vi "Fpga-Uart-State-Machine.vi"(5 "reset_rtl":bool, 6 "TX FIFO In":refnum<k21>="HT-UART_TX", 7 "RXD Pin In":refnum<k21>="UserRTL_d_microblaze_wrapper\\uart_rtl_rxd", 8 "RX FIFO In":refnum<k21>="TH-UART_RX", 9 "TXD Pin In":refnum<k21>="UserRTL_d_microblaze_wrapper\\uart_rtl_txd", 10 "Baud Rate":u32(ring)=128000 items=["110"=110, "300"=300, "1200"=1200, "2400"=2400, "4800"=4800, "9600"=9600, "19200"=19200, "38400"=38400, "57600"=57600, "115200"=115200, "128000"=128000, "230400"=230400, "460800"=460800, "921600"=921600], 11 "FPGA Clock Rate (MHz)":u32=100) -> ()   [LabVIEW 2017]
uses:
  <vilib>/Platform/TimedLoop/XDataNode/timing_clust.ctl
  <vilib>/Platform/TimedLoop/XDataNode/nitl_modes.ctl
  <vilib>/Platform/TimedLoop/XDataNode/wakeup.ctl
  UART.RX.States.2.ctl
  UART.RX.States.ctl
  <vilib>/rvi/Emulation/niFpgaSctlEmulationGetInTimedLoop.vi
  <vilib>/rvi/Emulation/niFpgaEmulationReportErrorSimple.vi
  <vilib>/rvi/Emulation/niFpgaGetClockAttributes.vi
  <vilib>/rvi/Emulation/niFpgaCriticalErrorInLSC.vi
  <vilib>/rvi/eio/common/nirviEmuTemplateMethod_errors.vi
  <vilib>/rvi/DataTransferAndStorage/Container/Common/niFpgaContainerExecOnDevCompGetState.vi
  <vilib>/rvi/Emulation/niFpgaEmulationIsFPGAContextNoSignature.vi
  <vilib>/rvi/errors/niFpgaSetErrorForExecOnDevCompSimple.vi
  <vilib>/rvi/eio/common/nirviEmuReportErrorAndStop.vi
  <vilib>/rvi/DataTransferAndStorage/Container/Common/niFpgaContainerGetUniqueNameForEmu.vi
  <vilib>/rvi/FIFO/Fifo_Resource/nirvififoEmulationSetSize.vi
  <vilib>/rvi/FIFO/Fifo_Resource/nirviFifoEmulationQueueMgr.vi
  <instcachedir>/0/nirviFifoEmulationQueueMgr_E5CAEC123FF24DC58D834DCA3CDAA9B5.lvgen/nirviFifoEmulationQueueMgr_E5CAEC123FF24DC58D834DCA3CDAA9B5_004.vi
  <vilib>/rvi/FIFO/Fifo_Resource/nirvififoEmulationDetermineInputValidOut.vi
  <vilib>/rvi/FIFO/Fifo_Resource/nirvififoEmulationCreateLock.vi
  <vilib>/rvi/Emulation/niFpgaProcessEmulError.vi
  <vilib>/rvi/FIFO/Fifo_Resource/nirvififoEmulationObtainLock.vi
  <vilib>/rvi/FIFO/Fifo_Resource/nirvififoEmulationReleaseLock.vi
  <vilib>/rvi/occurrence/nirviWaitOnOccurrenceBase.vi
  <vilib>/rvi/errors/nirviReportUnexpectedCaseInternalError.vi
  <vilib>/rvi/errors/nirviReportUnexpectedCaseInternalError (U32).vi
  <vilib>/Utility/error.llb/Clear Errors.vi
  <vilib>/rvi/interface/RandomDataEmulation/niFpgaRandomDataHandleErrors.vi
  <vilib>/Platform/TimedLoop/XDataNode/XDataNode.xnode
  <vilib>/eio/EIONode/EIONode.xnode
  <vilib>/rvi/DataTransferAndStorage/Container/XNode/niFpgaContainer.xnode
  <vilib>/rvi/FIFO/Fifo_Resource/niFpgaFifoEmulationRefIn.vi
  <vilib>/Platform/TimedLoop/XDataNode/XDNodeRunTimeDep.lvlib
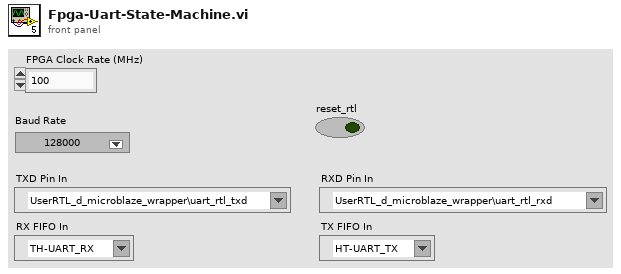
[diagram p1: front panel]
types:
  T1 = typedef "XDNodeRunTimeDep.lvlib/timing_clust.ctl" = cluster{"Expected End [f-1]":u64, "Actual End [f-1]":u64, "Finished Late? [f-1]":bool, "Expected End [i-1]":u64, "Actual End [i-1]":u64, "Finished Late? [i-1]":bool, "Expected Start [i]":u64, "Actual Start [i]":u64, "Expected Start [f]":u64, "Actual Start [f]":u64, "Source Name":string, "Structure Name":string, "Period":i64, "Deadline":i64, "Offset":i64, "Start":i64, "Priority":i32, "Timeout":i32, "Mode":T2, "Wakeup Reason":T3, "Error":errorcluster, "Source Type":string, "Secondary Source Type":string, "Global End Time":u64, "Global Start Time":u64, "Frame Duration":u64, "Iteration Duration":u64, "Assigned CPU":i32, "I/O Scan Engine Mode":u32}
  T2 = typedef "XDNodeRunTimeDep.lvlib/nitl_modes.ctl" = enum32{"No Change", "Process missed periods, maintain original phase", "Discard missed periods, maintain original phase", "Process missed periods, ignore original phase", "Discard missed periods, ignore original phase"}
  T3 = typedef "XDNodeRunTimeDep.lvlib/wakeup.ctl" = enum32{"Normal", "Aborted", "Asynchronous wakeup", "Timing source error", "Timed loop error", "Timeout"}
  T4 = typedef "UART.RX.States.2.ctl" = enum16{"No-Wait", "Wait-Half", "Wait-Full", "Wait-One-and-a-Half"}
  T5 = typedef "UART.RX.States.ctl" = enum16{"Read-StartBit", "Read-DataBits", "Read-Parity", "Read-StopBit", "Shift"}
  T6 = enum16{"Wait.for.New", "Send.StartBit", "Send.DataBits", "Send.Parity", "Send.StopBit"}
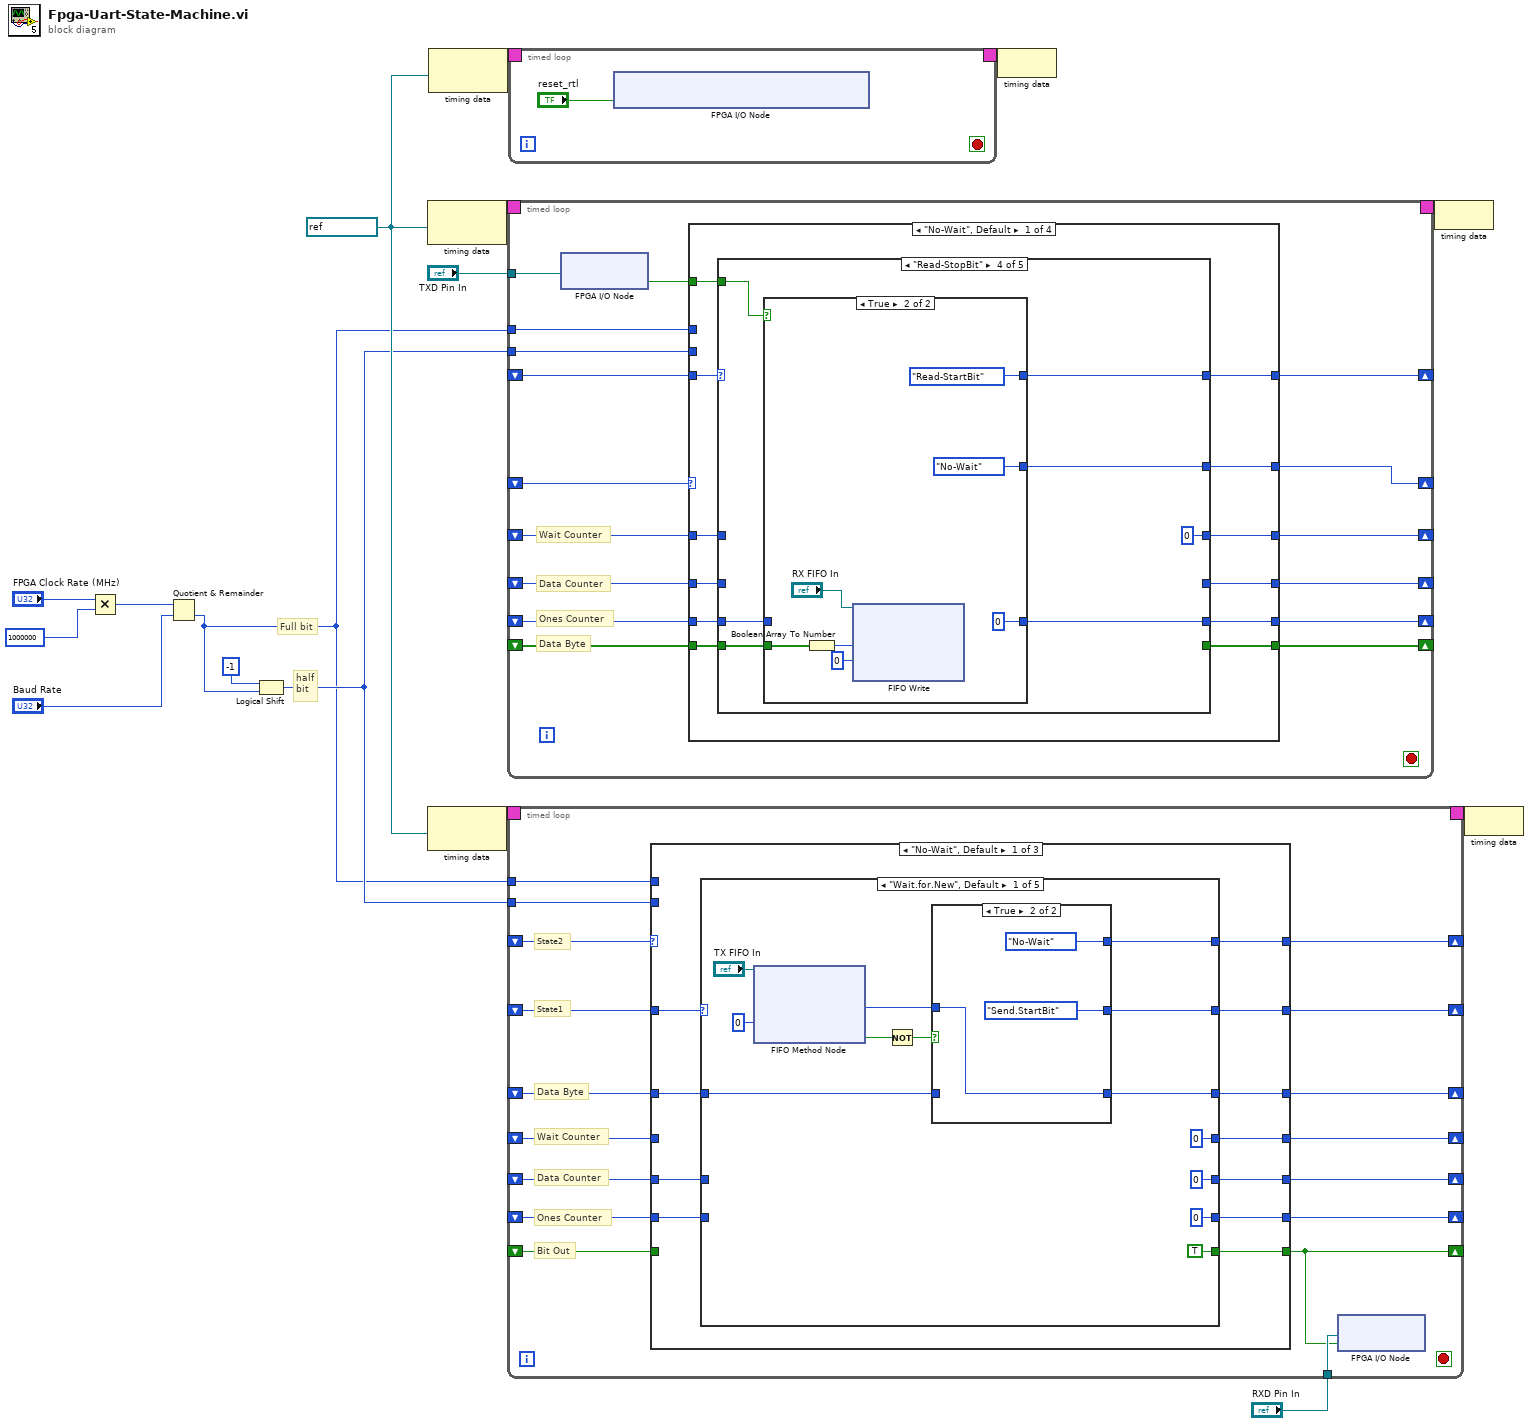
[diagram p0: block diagram]
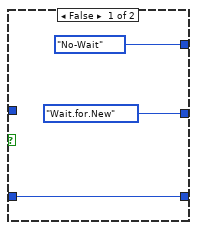
[diagram p2: hidden frame]
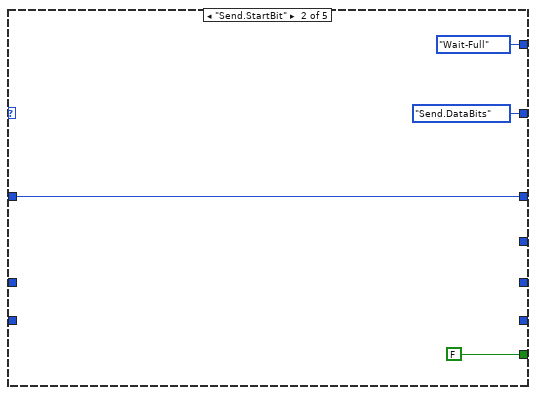
[diagram p3: hidden frame]
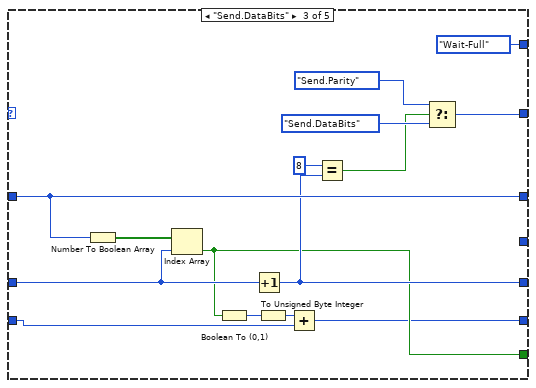
[diagram p4: hidden frame]
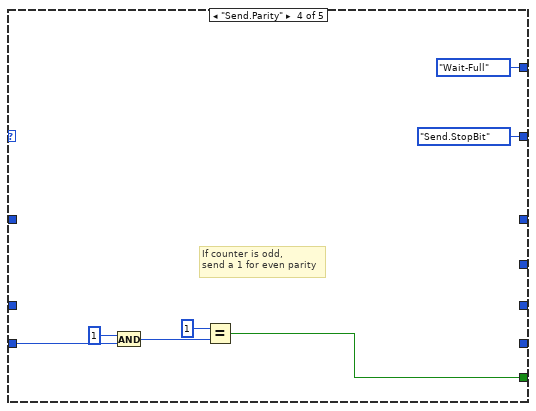
[diagram p5: hidden frame]
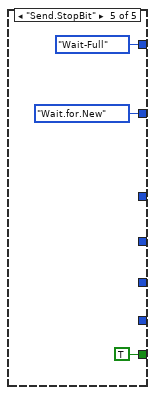
[diagram p6: hidden frame]
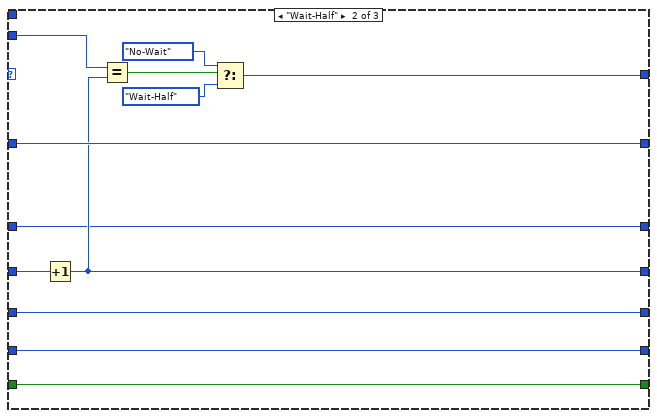
[diagram p7: hidden frame]
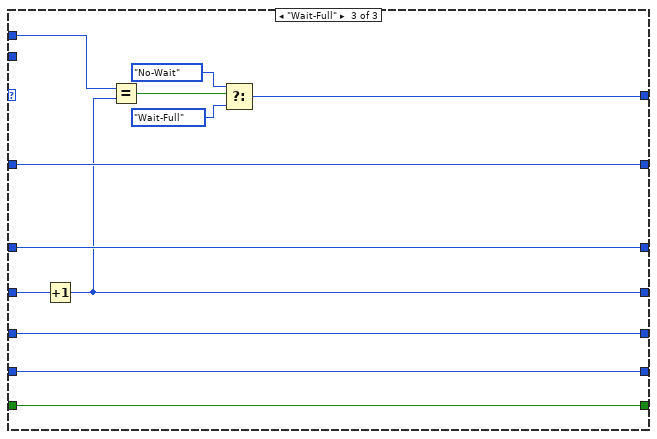
[diagram p8: hidden frame]
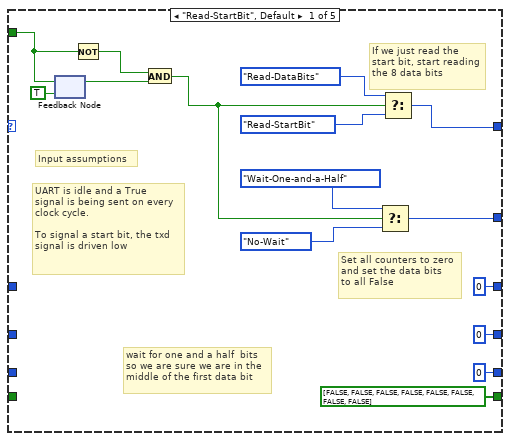
[diagram p9: hidden frame]
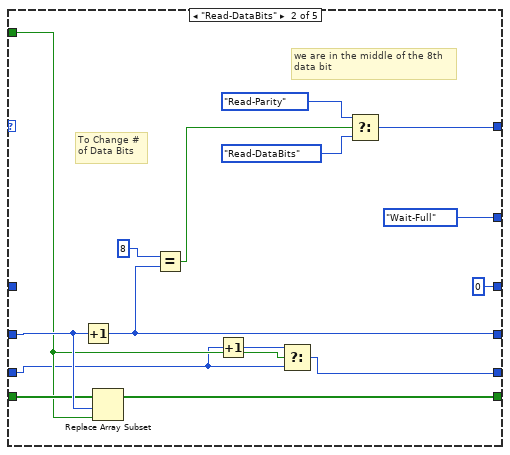
[diagram p10: hidden frame]
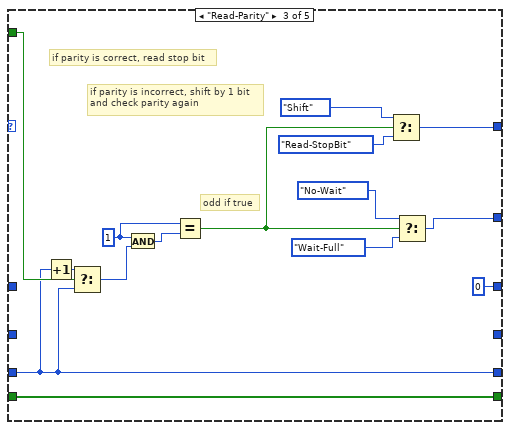
[diagram p11: hidden frame]
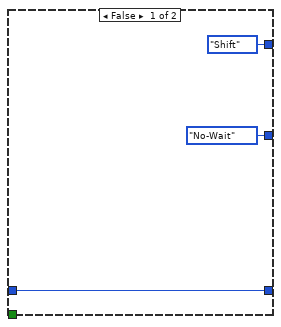
[diagram p12: hidden frame]
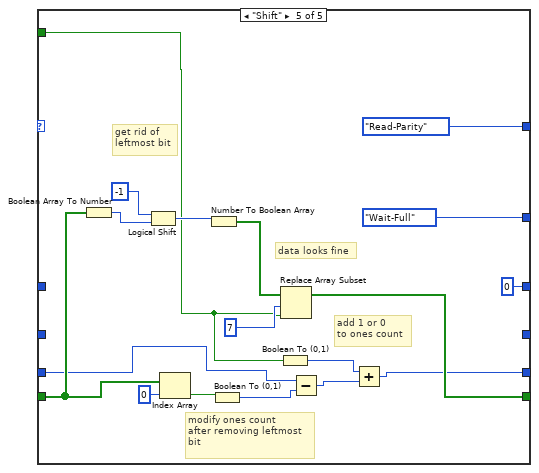
[diagram p13: hidden frame]
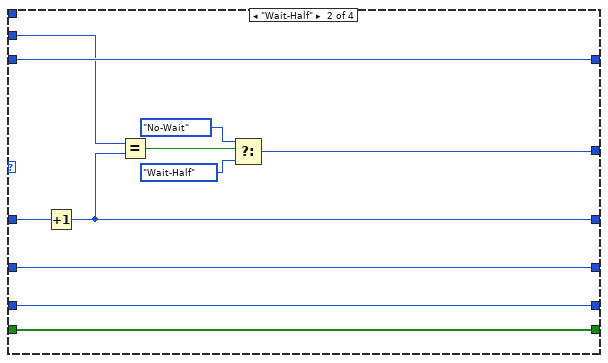
[diagram p14: hidden frame]
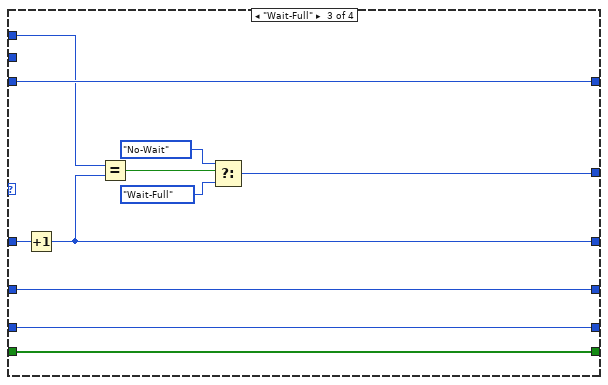
[diagram p15: hidden frame]
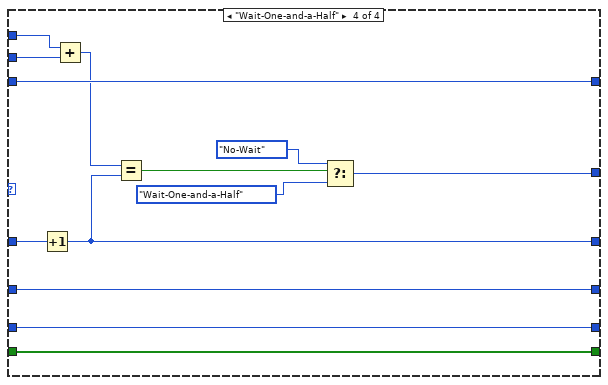
[diagram p16: hidden frame]
diagram:
  w3 = refnum<k21> "100MHz" ("Source Name")
  # "half\nbit"
  # "Full bit"
  n1 = Multiply(x="FPGA Clock Rate (MHz)", y=u32 1000000) -> (x*y=w15:u32)
  n2 = Quotient & Remainder(x=w15, y="Baud Rate") -> (floor(x/y)=w1:u32)  [unwired: 1 out]
  n3 = Logical Shift(y=i16 -1, x=w1) -> (x << y=w2:u32)
  n4 = node-c288(w3) -> (w10:T1)
  n5 = node-c288(w3) -> (w6:T1)
  n6 = node-c288(w3) -> (w12:T1)
  n7 = timed-loop {
    timing: w10 -> [_]
    timing-out: [_] -> w9
    shift-right: [w31] -> _
    shift-left: _ -> [w32]
    shift-right: [w29] -> _
    shift-left: _ -> [w30]
    shift-right: [w26] -> _
    shift-left: _ -> [w28]
    shift-right: [w25] -> _
    shift-left: _ -> [w27]
    tunnel: w1 -> [w24]
    tunnel: w2 -> [w23]
    shift-right: [w22] -> _
    shift-left: _ -> [w21]
    shift-right: [w19] -> _
    shift-left: _ -> [w20]
    tunnel: "TXD Pin In" -> [w18]
    stop <- _ stop-if-true
    # "Data Byte"
    # "Ones Counter"
    # "Data Counter"
    # "Wait Counter"
    n8 = xnode "FPGA I/O Node"("FPGA I/O In"=w18) -> ("I/O Item"=w17:bool)  [unwired: 1 out]
    n9 = case shown="\"No-Wait\", Default" w30 {
      tunnel: w32 -> [w40 w129 w138 w151]
      tunnel: w17 -> [w33 _ _ _]
      tunnel: [w39 w129 w138 w151] -> w31
      tunnel: [w38 w130 w142 w155] -> w29
      tunnel: w28 -> [w44 w135 w143 w156]
      tunnel: w27 -> [w43 w128 w141 w154]
      tunnel: [w37 w134 w140 w153] -> w26
      tunnel: [w36 w128 w141 w154] -> w25
      tunnel: w24 -> [_ _ w137 w149]
      tunnel: w23 -> [_ w126 _ w148]
      tunnel: [w34 w127 w139 w152] -> w22
      tunnel: w21 -> [w42 w127 w139 w152]
      tunnel: w20 -> [w41 w125 w136 w150]
      tunnel: [w35 w125 w136 w150] -> w19
      frame "No-Wait", Default {
        n10 = case shown="\"Read-StopBit\"" w40 {
          tunnel: w33 -> [w56 w64 w89 w95 w111]
          tunnel: [w55 w65 w85 w93 UART.RX.States."Read-Parity"] -> w39
          tunnel: [w49 UART.RX.States.2."Wait-Full" w80 w94 UART.RX.States.2."Wait-Full"] -> w38
          tunnel: w44 -> [_ _ _ _ _]
          tunnel: w43 -> [_ w73 _ _ _]
          tunnel: [u32 0 ("Wait Counter") u32 0 ("Wait Counter") u32 0 ("Wait Counter") u32 0 ("Wait Counter") u32 0 ("Wait Counter")] -> w37
          tunnel: [u32 0 ("Data Counter") w70 _ _ _] -> w36
          tunnel: [bool[] [FALSE, FALSE, FALSE, FALSE, FALSE, FALSE, FALSE, FALSE] w71 w78 _ w117] -> w34
          tunnel: w42 -> [_ w72 w78 w96 w116]
          tunnel: w41 -> [_ w63 w76 w91 w114]
          tunnel: [u32 0 ("Data Counter") w61 w76 w92 w109] -> w35
          frame "Read-StartBit", Default {
            # "Set all counters to zero\nand set the data bits\nto all False"
            # "wait for one and a half  bits\nso we are sure we are in the\nmiddle of the first data bit"
            # "If we just read the \nstart bit, start reading\nthe 8 data bits"
            # "UART is idle and a True\nsignal is being sent on every\nclock cycle.\n\nTo signal a start bit, the txd\nsignal is driven low"
            # "Input assumptions"
            n11 = feedback #1(TRUE ("d_microblaze_i\\uart_rtl_txd")) -> (w59:bool)
            n12 = feedback-in #1(w56) -> ()
            n13 = Not(x=w56) -> (.not. x?=w58:bool)
            n14 = And(x=w58, y=w59) -> (x .and. y?=w52:bool)
            n15 = Select(t=UART.RX.States.2."Wait-One-and-a-Half", s=w52, f=UART.RX.States.2."No-Wait") -> (s? t:f=w49:T4)
            n16 = Select(t=UART.RX.States."Read-DataBits", s=w52, f=UART.RX.States."Read-StartBit") -> (s? t:f=w55:T5)
          }
          frame "Read-DataBits" {
            # "we are in the middle of the 8th\ndata bit"
            # "To Change #\nof Data Bits"
            n17 = Increment(x=w73) -> (x+1=w70:u32)
            n18 = Replace Array Subset(array=w72, new element=w64, index=w73) -> (w71:bool[])
            n19 = Equal?(x=u32 8, y=w70) -> (x = y?=w68:bool)
            n20 = Increment(x=w63) -> (x+1=w62:u32)
            n21 = Select(t=w62, s=w64, f=w63) -> (s? t:f=w61:u32)
            n22 = Select(t=UART.RX.States."Read-Parity", s=w68, f=UART.RX.States."Read-DataBits") -> (s? t:f=w65:T5)
          }
          frame "Read-Parity" {
            w86 = u32 1 ("x")
            # "odd if true"
            # "if parity is incorrect, shift by 1 bit\nand check parity again"
            # "if parity is correct, read stop bit"
            n23 = Increment(x=w76) -> (x+1=w88:u32)
            n24 = Select(t=w88, s=w89, f=w76) -> (s? t:f=w77:u32)
            n25 = And(x=w86, y=w77) -> (x .and. y?=w87:u32)
            n26 = Equal?(x=w86, y=w87) -> (x = y?=w82:bool)
            n27 = Select(t=UART.RX.States."Shift", s=w82, f=UART.RX.States."Read-StopBit") -> (s? t:f=w85:T5)
            n28 = Select(t=UART.RX.States.2."No-Wait", s=w82, f=UART.RX.States.2."Wait-Full") -> (s? t:f=w80:T4)
          }
          frame "Read-StopBit" {
            n29 = case shown="True" w95 {
              tunnel: w96 -> [_ w104]
              tunnel: [UART.RX.States.2."No-Wait" UART.RX.States.2."No-Wait"] -> w94
              tunnel: [UART.RX.States."Shift" UART.RX.States."Read-StartBit"] -> w93
              tunnel: [w97 u32 0 ("Ones Counter")] -> w92
              tunnel: w91 -> [w97 _]
              frame False {
              }
              frame True {
                n30 = Boolean Array To Number(Boolean array=w104) -> (number=w106:u8)
                n31 = xnode ("FIFO Write")("Element"=w106, "Timeout"=0, "FIFO In"="RX FIFO In") -> ()  [unwired: 2 out]
              }
            }
          }
          frame "Shift" {
            # "data looks fine"
            # "add 1 or 0\nto ones count"
            # "modify ones count\nafter removing leftmost\nbit"
            # "get rid of\nleftmost bit"
            n32 = Boolean Array To Number(Boolean array=w116) -> (number=w124:u8)
            n33 = Logical Shift(y=i16 -1, x=w124) -> (x << y=w122:u8)
            n34 = Index Array(array=w116, index=0) -> (element=w115:bool)
            n35 = Number To Boolean Array(number=w122) -> (Boolean array=w119:bool[])
            n36 = Boolean To (0,1)(Boolean=w115) -> (0, 1=w113:i16)
            n37 = Boolean To (0,1)(Boolean=w111) -> (0, 1=w110:i16)
            n38 = Replace Array Subset(array=w119, new element=w111, index=7) -> (w117:bool[])
            n39 = Subtract(x=w114, y=w113) -> (x-y=w112:u32)
            n40 = Add(x=w110, y=w112) -> (x+y=w109:u32)
          }
        }
      }
      frame "Wait-Half" {
        n41 = Increment(x=w135) -> (x+1=w134:u32)
        n42 = Equal?(x=w126, y=w134) -> (x = y?=w133:bool)
        n43 = Select(t=UART.RX.States.2."No-Wait", s=w133, f=UART.RX.States.2."Wait-Half") -> (s? t:f=w130:T4)
      }
      frame "Wait-Full" {
        n44 = Increment(x=w143) -> (x+1=w140:u32)
        n45 = Equal?(x=w137, y=w140) -> (x = y?=w146:bool)
        n46 = Select(t=UART.RX.States.2."No-Wait", s=w146, f=UART.RX.States.2."Wait-Full") -> (s? t:f=w142:T4)
      }
      frame "Wait-One-and-a-Half" {
        n47 = Increment(x=w156) -> (x+1=w153:u32)
        n48 = Add(x=w149, y=w148) -> (x+y=w147:u32)
        n49 = Equal?(x=w147, y=w153) -> (x = y?=w159:bool)
        n50 = Select(t=UART.RX.States.2."No-Wait", s=w159, f=UART.RX.States.2."Wait-One-and-a-Half") -> (s? t:f=w155:T4)
      }
    }
  }
  n51 = timed-loop {
    timing: w6 -> [_]
    timing-out: [_] -> w5
    shift-right: [w173] -> _
    shift-left: _ -> [w177]
    shift-right: [w176] -> _
    shift-left: _ -> [w178]
    shift-right: [w175] -> _
    shift-left: _ -> [w174]
    shift-right: [w172] -> _
    shift-left: _ -> [w171]
    tunnel: w2 -> [w170]
    tunnel: w1 -> [w169]
    tunnel: "RXD Pin In" -> [w168]
    shift-right: [w167] -> _
    shift-left: _ -> [w166]
    shift-right: [w165] -> _
    shift-left: _ -> [w164]
    shift-right: [w163] -> _
    shift-left: _ -> [w162]
    stop <- _ stop-if-true
    # "Ones Counter"
    # "Bit Out"
    # "Data Counter"
    # "Data Byte"
    # "State1"
    # "State2"
    # "Wait Counter"
    n52 = case shown="\"No-Wait\", Default" w177 {
      tunnel: w178 -> [w189 w243 w255]
      tunnel: [w188 w243 w255] -> w176
      tunnel: [w187 w239 w253] -> w175
      tunnel: w174 -> [w186 w239 w253]
      tunnel: [w185 w246 w258] -> w173
      tunnel: [w184 w240 w252] -> w172
      tunnel: w171 -> [_ w245 w257]
      tunnel: w170 -> [_ w244 _]
      tunnel: w169 -> [_ _ w256]
      tunnel: [w183 w242 w254] -> w167
      tunnel: w166 -> [_ w242 w254]
      tunnel: [w182 w241 w251] -> w165
      tunnel: w164 -> [w181 w241 w251]
      tunnel: [w180 w238 w250] -> w163
      tunnel: w162 -> [w179 w238 w250]
      frame "No-Wait", Default {
        n53 = case shown="\"Wait.for.New\", Default" w189 {
          tunnel: [w198 T6."Send.DataBits" w220 T6."Send.StopBit" T6."Wait.for.New"] -> w188
          tunnel: [w196 w209 w225 _ _] -> w187
          tunnel: w186 -> [w194 w209 w225 _ _]
          tunnel: [w197 UART.RX.States.2."Wait-Full" UART.RX.States.2."Wait-Full" UART.RX.States.2."Wait-Full" UART.RX.States.2."Wait-Full"] -> w185
          tunnel: [u32 0 ("Wait Counter") _ _ _ _] -> w184
          tunnel: [TRUE ("I/O Item") FALSE ("I/O Item") w217 w228 TRUE ("I/O Item")] -> w183
          tunnel: [u8 0 ("Wait Counter") _ w223 _ _] -> w182
          tunnel: w181 -> [_ _ w226 _ _]
          tunnel: [u8 0 ("Wait Counter") _ w216 _ _] -> w180
          tunnel: w179 -> [_ _ w214 w232 _]
          frame "Wait.for.New", Default {
            n54 = xnode ("FIFO Method Node")("Timeout"=0, "FIFO In"="TX FIFO In") -> ("Element"=w195:u8, "Timed Out?"=w200:bool)  [unwired: 1 out]
            n55 = Not(x=w200) -> (.not. x?=w199:bool)
            n56 = case shown="True" w199 {
              tunnel: [T6."Wait.for.New" T6."Send.StartBit"] -> w198
              tunnel: [UART.RX.States.2."No-Wait" UART.RX.States.2."No-Wait"] -> w197
              tunnel: [w203 w206] -> w196
              tunnel: w195 -> [_ w206]
              tunnel: w194 -> [w203 _]
              frame False {
              }
              frame True {
              }
            }
          }
          frame "Send.StartBit" {
          }
          frame "Send.DataBits" {
            n57 = Number To Boolean Array(number=w225) -> (Boolean array=w227:bool[])
            n58 = Index Array(array=w227, index=w226) -> (element=w217:bool)
            n59 = Boolean To (0,1)(Boolean=w217) -> (0, 1=w215:i16)
            n60 = Increment(x=w226) -> (x+1=w223:u8)
            n61 = To Unsigned Byte Integer(number=w215) -> (unsigned 8bit integer=w213:u8)
            n62 = Add(x=w213, y=w214) -> (x+y=w216:u8)
            n63 = Equal?(x=u8 8, y=w223) -> (x = y?=w219:bool)
            n64 = Select(t=T6."Send.Parity", s=w219, f=T6."Send.DataBits") -> (s? t:f=w220:T6)
          }
          frame "Send.Parity" {
            # "If counter is odd,\nsend a 1 for even parity"
            n65 = And(x=i16 1, y=w232) -> (x .and. y?=w230:i16)
            n66 = Equal?(x=i16 1, y=w230) -> (x = y?=w228:bool)
          }
          frame "Send.StopBit" {
          }
        }
      }
      frame "Wait-Half" {
        n67 = Increment(x=w245) -> (x+1=w240:u32)
        n68 = Equal?(x=w244, y=w240) -> (x = y?=w249:bool)
        n69 = Select(t=UART.RX.States.2."No-Wait", s=w249, f=UART.RX.States.2."Wait-Half") -> (s? t:f=w246:T4)
      }
      frame "Wait-Full" {
        n70 = Increment(x=w257) -> (x+1=w252:u32)
        n71 = Equal?(x=w256, y=w252) -> (x = y?=w261:bool)
        n72 = Select(t=UART.RX.States.2."No-Wait", s=w261, f=UART.RX.States.2."Wait-Full") -> (s? t:f=w258:T4)
      }
    }
    n73 = xnode "FPGA I/O Node"("I/O Item"=w167, "FPGA I/O In"=w168) -> ()  [unwired: 1 out]
  }
  n74 = timed-loop {
    timing: w12 -> [_]
    timing-out: [_] -> w11
    stop <- _ stop-if-true
    n75 = xnode "FPGA I/O Node"("UserRTL_d_microblaze_wrapper\\reset_rtl"="reset_rtl") -> ()  [unwired: 1 in, 1 out]
  }
  n76 = node-c288(w11) -> ()
  n77 = node-c288(w9) -> ()
  n78 = node-c288(w5) -> ()
